vi "Close.vi"(8 "error in (no error)":errorcluster, 10 "Msg in":T1, 11 "FakePressureController in":refnum<class "MagAnalysis_Online.lvclass">) -> (0 "error out":errorcluster, 1 "new command":string, 2 "Msg out":T1, 3 "FakePressureController out":refnum<class "MagAnalysis_Online.lvclass">)   [LabVIEW 2011, in "MagAnalysis_Online.lvclass"]
uses:
  MagAnalysis_Online.lvclass
  DriverMsg.ctl
  BaseDriver/BaseDriver.lvclass
  MagAnalysis_Online.lvclass/MagAnalysis_Online.ctl
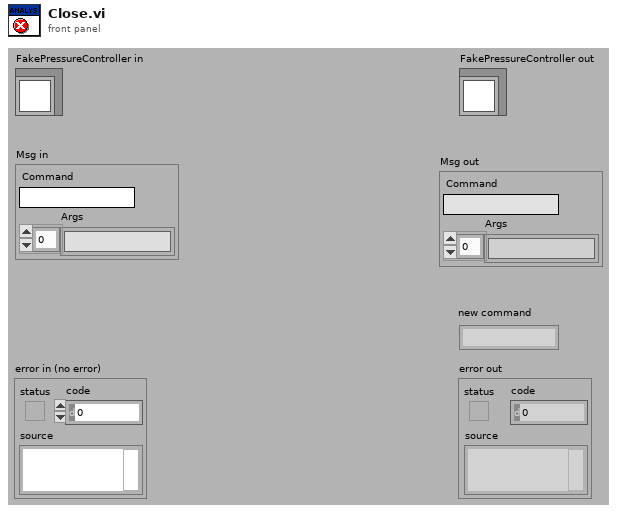
[diagram p1: front panel]
types:
  T1 = typedef "DriverMsg.ctl" = cluster{"Command":string, "Args":string[]}
  T2 = typedef "IMAQ Image.ctl" = refnum<image>
  T3 = typedef "MagAnalysis_Online.lvclass/analysis_data_typdef.ctl" = cluster{"cam0":T2, "cam1":T2, "cam2":T2, "cam3":T2}
  T4 = typedef "bgImages_tyudef.ctl" = cluster{"cam 0":T2, "cam 1":T2, "cam 2":T2, "cam 3":T2}
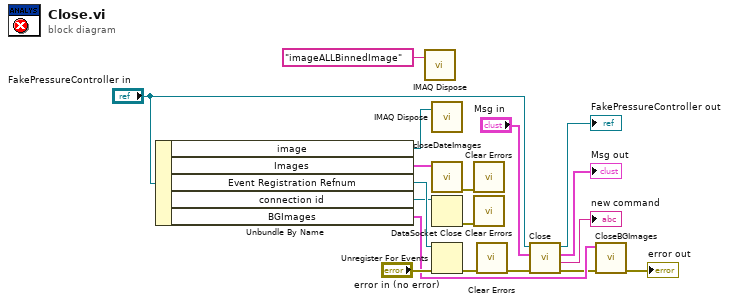
[diagram p0: block diagram]
diagram:
  n1 = Unbundle By Name("FakePressureController in") -> ("image"=w4:T2, "Images"=w1:T3, "Event Registration Refnum"=w13:refnum<event-registration>, "connection id"=w9:refnum<k13>, "BGImages"=w7:T4)
  n2 = call "IMAQ Dispose"("Image"="imageALLBinnedImage" ("Image Name")) -> ()  [unwired: 5 in, 1 out]
  n3 = call "IMAQ Dispose"("Image"=w4) -> ()  [unwired: 5 in, 1 out]
  n4 = call "closeDateImages.vi"("data"=w1) -> ("error out"=w2:errorcluster)  [unwired: 10 in]
  n5 = DataSocket Close(11:w9) -> (0:w8:errorcluster)  [unwired: 2 in, 1 out]
  n6 = Unregister For Events(event registration refnum=w13, error in="error in (no error)") -> (error out=w10:errorcluster)
  n7 = call "Clear Errors.vi"("error in (no error)"=w2) -> ()  [unwired: 6 in, 1 out]
  n8 = call "Clear Errors.vi"("error in (no error)"=w8) -> ()  [unwired: 6 in, 1 out]
  n9 = call "Clear Errors.vi"("error in (no error)"=w10) -> ("error out"=w11:errorcluster)  [unwired: 6 in]
  n10 = call-parent "Close.vi"("error in (no error)"=w11, "Msg in"="Msg in", "BaseDriver in"="FakePressureController in") -> ("error out"=w6:errorcluster, "new command"=→"new command":string, "Msg out"=→"Msg out":T1, "BaseDriver out"=→"FakePressureController out":refnum<class "MagAnalysis_Online.lvclass">)  [unwired: 5 in]
  n11 = call "CloseBGImages.vi"("error in (no error)"=w6, "BGImages"=w7) -> ("error out"=→"error out":errorcluster)  [unwired: 9 in]
